vi "clearpath_enqueue_xmitqueue.vi"(0 "ClearpathComm":T1, 1 "Cluster":cluster{"buf":u8[], "return type":i32, i32}) -> ()   [LabVIEW 2010, in "clearpath_interface.lvlib"]
uses:
  clearpath_interface.lvlib
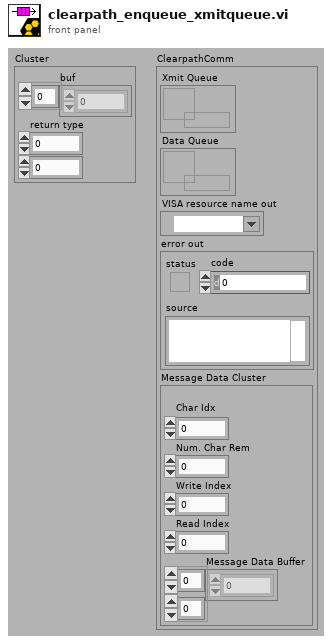
[diagram p1: front panel]
types:
  T1 = cluster{"Xmit Queue":refnum<queue>, "Data Queue":refnum<queue>, "VISA resource name out":refnum<visa-resource-name>, "error out":errorcluster, "Message Data Cluster":cluster{"\nChar Idx":u8, "Num. Char Rem":u8, "Write Index":u8, "Read Index":u8, "Message Data Buffer":u8[][]}}
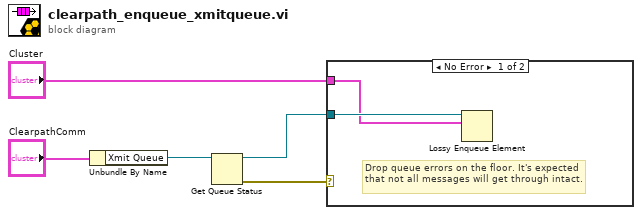
[diagram p0: block diagram]
diagram:
  n1 = Unbundle By Name("ClearpathComm") -> ("Xmit Queue"=w2:refnum<queue>)
  n2 = Get Queue Status(queue=w2) -> (queue out=w3:refnum<queue>, error out=w4:errorcluster)  [unwired: 2 in, 6 out]
  n3 = case shown="No Error" w4 {
    tunnel: w3 -> [w7 _]
    tunnel: "Cluster" -> [w6 _]
    frame No Error {
      # "Drop queue errors on the floor. It's expected that not all messages will get through intact."
      n4 = Lossy Enqueue Element(queue=w7, element=w6) -> ()  [unwired: 1 in, 4 out]
    }
    frame Error {
    }
  }
